vi "lvpeak_get_last_error.vi"() -> (2 "message":string, 3 "code":u32)   [LabVIEW 2024, in "Vision.lvlib"]
uses:
  Vision.lvlib
  bin/LVPeak.dll
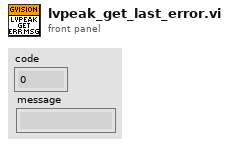
[diagram p1: front panel]
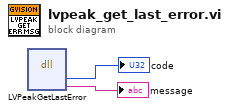
[diagram p0: block diagram]
diagram:
  n1 = dll-call lib="C:/Users/cfang/Desktop/nebraska-silicon-lab/pixel-gantry-control/Gantry/Shared Components/bin/LVPeak.dll" fn="LVPeakGetLastError"() -> ("code"=→"code":u32, "message"=→"message":string)  [unwired: 6 in, 2 out]
